vi "AFG3352X.get library version.vi"() -> (0 "nameAndVersion":string)   [LabVIEW 2014, in "AFG3352X.lvlib"]
doc: "obtain name and version of a library as a string"
uses:
  AFG3352X.lvlib
  CSlibraries/UtilityLib/UtilityLib.lvlib
  instr.lib/Agilent 3352X Series/Agilent 3352X Series.lvlib
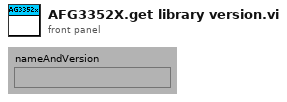
[diagram p1: front panel]
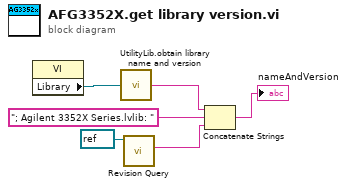
[diagram p0: block diagram]
diagram:
  n1 = property class="VI"() -> ("Library"=w6:refnum<vi>)  [unwired: 2 in, 2 out]
  n2 = call "UtilityLib.obtain library name and version.vi"("Library"=w6) -> ("nameAndVersion"=w4:string)
  n3 = call "Revision Query.vi"("VISA resource name"=refnum<visa-resource-name> refnum) -> ("Instrument Driver Revision"=w3:string)  [unwired: 7 in, 3 out]
  n4 = Concatenate Strings(w4, "; Agilent 3352X Series.lvlib: " ("string"), w3) -> (→"nameAndVersion":string)
